vi "Replace Single Overlay.vi"(6 "Show Text":bool, 8 "error in":errorcluster, 10 "Litho":T2, 11 "BigMAQ in":refnum<class "BigMAQ.lvclass">) -> (0 "error out":errorcluster, 3 "BigMAQ out":refnum<class "BigMAQ.lvclass">)   [LabVIEW 2019, in "BigMAQ.lvclass"]
uses:
  BigMAQ.lvclass
  <userlib>/LevyLab/Relay Box/Typedefs/Resistor--enum.ctl
  Overlay.ctl
  BigMAQ.lvclass/BigMAQ.ctl
  <userlib>/LevyLab/Relay Box/Relay-Box.lvclass
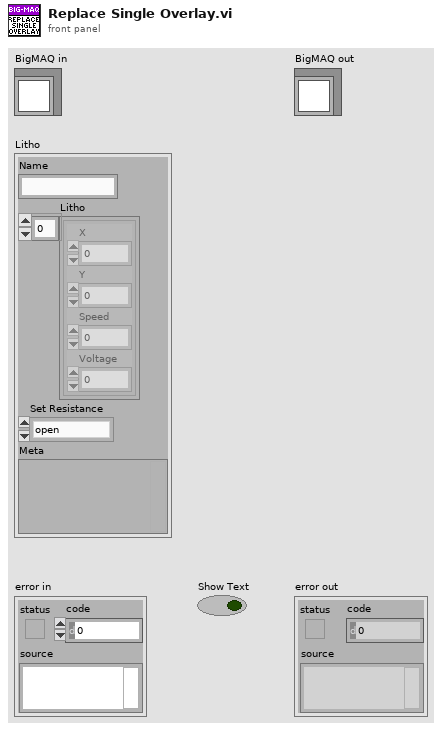
[diagram p1: front panel]
types:
  T1 = typedef "Relay-Box.lvclass/Resistor--enum.ctl" = enum16{"open", "discharge tip", "0 ohms", "100k ohm", "10M ohm", "1G ohm"}
  T2 = cluster{"Name":string, "Litho":cluster{"X":dbl, "Y":dbl, "Speed":dbl, "Voltage":dbl}[], "Set Resistance":T1, "Meta":variant}
  T3 = typedef "BigMAQ.lvclass/Overlay.ctl" = cluster{"Name":string, "Data":cluster{"Points":cluster{"X":dbl, "Y":dbl}[], "Voltages":dbl[]}, "Changes":cluster{"MD5 Digest":string, "Changed?":bool}}
  T4 = cluster{"X":dbl, "Y":dbl, "Speed":dbl, "Voltage":dbl}[]
  T5 = typedef "IMAQ Image.ctl" = refnum<image>
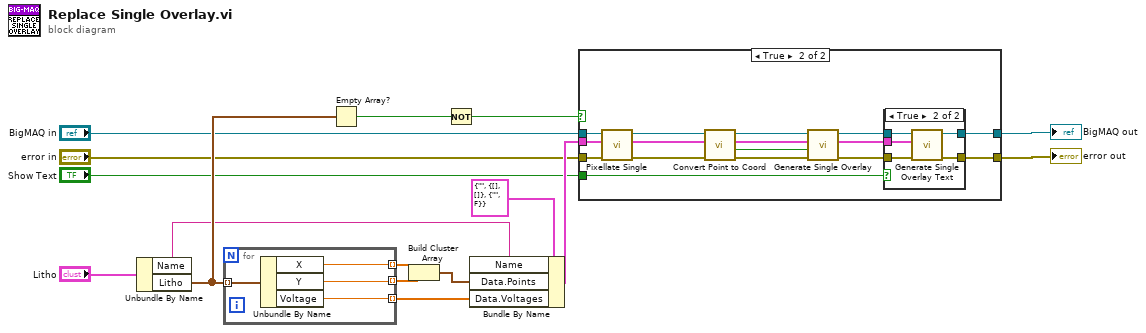
[diagram p0: block diagram]
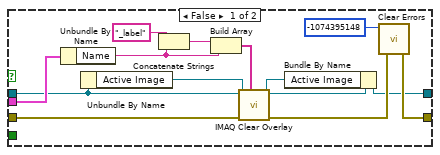
[diagram p2: hidden frame]
diagram:
  n1 = Unbundle By Name("Litho") -> ("Name"=w12:string, "Litho"=w14:T4)
  n2 = for {
    tunnel: w14 -> [w17] mode=indexing
    tunnel: [w20] -> w13 mode=indexing
    tunnel: [w19] -> w10 mode=indexing
    tunnel: [w18] -> w11 mode=indexing
    n3 = Unbundle By Name(w17) -> ("X"=w19:dbl, "Y"=w18:dbl, "Voltage"=w20:dbl)
  }
  n4 = Empty Array?(array=w14) -> (empty?=w15:bool)
  n5 = Build Cluster Array(w10, w11) -> (w9:cluster{"X":dbl, "Y":dbl}[])
  n6 = Not(x=w15) -> (.not. x?=w2:bool)
  n7 = Bundle By Name(cluster=T3 {"Name"="", "Data"={"Points"=[], "Voltages"=[]}, "Changes"={"MD5 Digest"="", "Changed?"=FALSE}} ("Overlay"), "Name"=w12, "Data.Points"=w9, "Data.Voltages"=w13) -> (w7:T3)
  n8 = case shown="True" w2 {
    tunnel: w7 -> [w31 w49]
    tunnel: "error in" -> [w33 w39]
    tunnel: [w24 w38] -> w5
    tunnel: "BigMAQ in" -> [w22 w37]
    tunnel: [w23 w36] -> w3
    tunnel: "Show Text" -> [_ w35]
    frame False {
      n9 = Unbundle By Name(w31) -> ("Name"=w27:string)
      n10 = Unbundle By Name(w22) -> ("Active Image"=w32:T5)
      n11 = Concatenate Strings("_label" ("string"), w27) -> (w29:string)
      n12 = Build Array(w29, w27) -> (w28:string[])
      n13 = call "IMAQ Clear Overlay"("Groups"=w28, "error in (no error)"=w33, "Image"=w32) -> ("error out"=w25:errorcluster, "Image Out"=w21:T5)  [unwired: 7 in]
      n14 = Bundle By Name(cluster=w22, "Active Image"=w21) -> (w23:refnum<class "BigMAQ.lvclass">)
      n15 = call <vilib>:"Clear Errors.vi"("error in (no error)"=w25, "specific error code to clear (0: all)"=-1074395148) -> ("error out"=w24:errorcluster)  [unwired: 4 in, 1 out]
    }
    frame True {
      n16 = call "Pixellate Single.vi"("error in"=w39, "Overlay"=w49, "BigMAQ in"=w37) -> ("error out"=w44:errorcluster, "Pixellated Overlay"=w48:T3, "BigMAQ out"=w45:refnum<class "BigMAQ.lvclass">)  [unwired: 6 in]
      n17 = call "Convert Point to Coord.vi"("error in"=w44, "Overlay"=w48, "BigMAQ in"=w45) -> ("error out"=w42:errorcluster, "Voltage Constant?"=w34:bool, "output cluster"=w47:T3, "BigMAQ out"=w43:refnum<class "BigMAQ.lvclass">)  [unwired: 5 in]
      n18 = call "Generate Single Overlay.vi"("error in"=w42, "Single Color"=w34, "Overlay"=w47, "BigMAQ in"=w43) -> ("error out"=w40:errorcluster, "Overlay Out"=w46:T3, "BigMAQ out"=w41:refnum<class "BigMAQ.lvclass">)  [unwired: 4 in, 1 out]
      n19 = case shown="True" w35 {
        tunnel: w46 -> [_ w56]
        tunnel: w41 -> [w51 w55]
        tunnel: w40 -> [w50 w54]
        tunnel: [w50 w53] -> w38
        tunnel: [w51 w52] -> w36
        frame False {
        }
        frame True {
          n20 = call "Generate Single Overlay Text.vi"("error in"=w54, "Overlay"=w56, "BigMAQ in"=w55) -> ("error out"=w53:errorcluster, "BigMAQ out"=w52:refnum<class "BigMAQ.lvclass">)  [unwired: 7 in]
        }
      }
    }
  }
  "error out" <- w5
  "BigMAQ out" <- w3
